vi "Test_temperature_read.vi"() -> ()   [LabVIEW 2019]
panel:
  out "Test array2_response":u8[](array[numeric])
  out "Test_array":u8[](array[numeric])
  out "Address response":u8
  out "String lenght test":i32
  out "raw command":u8
  in  "COM Port for serial\nconnection. Check device\nmanager.":string
  out "Decoded value":dbl
  out "Value response":i32
  out "Key response":u32
  in  "i2c address":u32
  in  "Address":u8
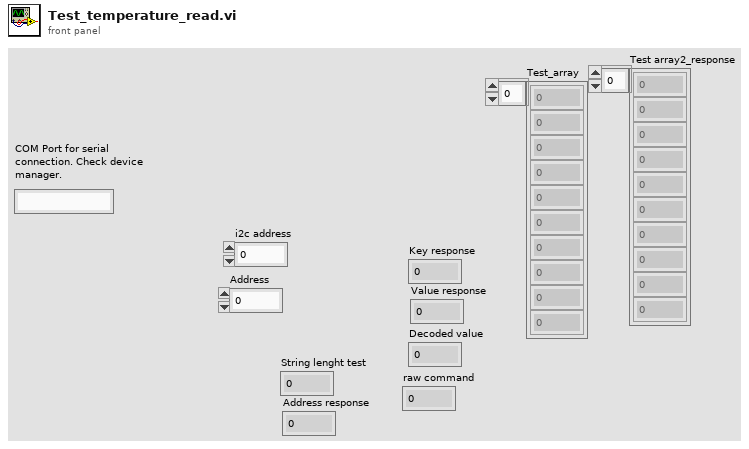
[diagram p1: front panel]
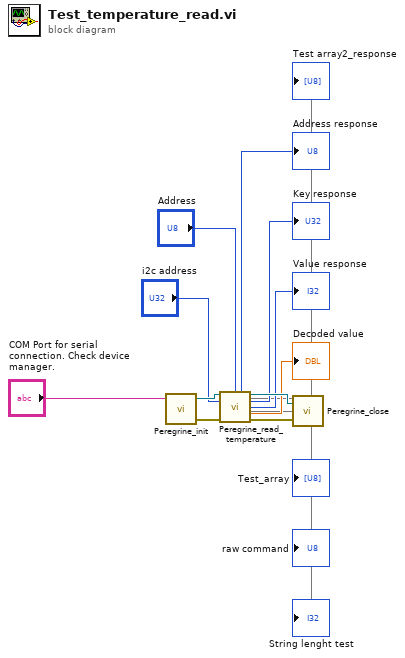
[diagram p0: block diagram]
diagram:
  n1 = call "Peregrine_init.vi"("COM Port for serial\nconnection. Check device\nmanager."="COM Port for serial\nconnection. Check device\nmanager.") -> ("error out"=w13:errorcluster, "Handle out"=w15:refnum<visa-resource-name>)  [unwired: 3 in]
  n2 = call "Peregrine_read_temperature.vi"("Handle in"=w15, "Address"="Address", "i2c address"="i2c address", "error"=w13) -> (1:→"Test array2_response", "Address response"=→"Address response":u8, "Handle out"=w14:refnum<visa-resource-name>, "Key response"=→"Key response":u32, "Value response"=→"Value response":i32, "Decoded value"=→"Decoded value":dbl, 12:→"String lenght test", 13:→"raw command", 14:→"Test_array", "error out"=w12:errorcluster)  [unwired: 2 in]
  n3 = call "Peregrine_close.vi"("error in (no error)"=w12, "Handle in"=w14) -> ()  [unwired: 1 in, 1 out]
